vi "CTRE_Phoenix_CANifier_SetControlFramePeriod.vi"(8 "error in (no error)":errorcluster, 9 "periodMs":i32, 10 "Pigeon IMU Control Frame":T1=272384 items=["CondStatus_Control_1"=272384], 11 "PigeonIMUDevRef":T2={"DeviceStatus"={"status"=FALSE, "code"=0, "source"=""}, "Device Number"=0, "Type"=352321536, "Device ID"=0, "Handle"=0, "UsageFrame"=0, "Library Path"=path ""} {"Type" items=["CAN"=352321536, "TalonSRX"=33554432]}) -> (0 "error out":errorcluster, 3 "PigeonIMUDevRef":T2={"DeviceStatus"={"status"=FALSE, "code"=0, "source"=""}, "Device Number"=0, "Type"=352321536, "Device ID"=0, "Handle"=0, "UsageFrame"=0, "Library Path"=path ""} {"Type" items=["CAN"=352321536, "TalonSRX"=33554432]})   [LabVIEW 2017]
doc: "Set the period of the specified control frame."
uses:
  CTRE_PigeonIMU_DeviceRef.ctl
  CTRE_PigeonIMU_ConnectionType.ctl
  CTRE_PigeonIMU_ControlFrame.ctl
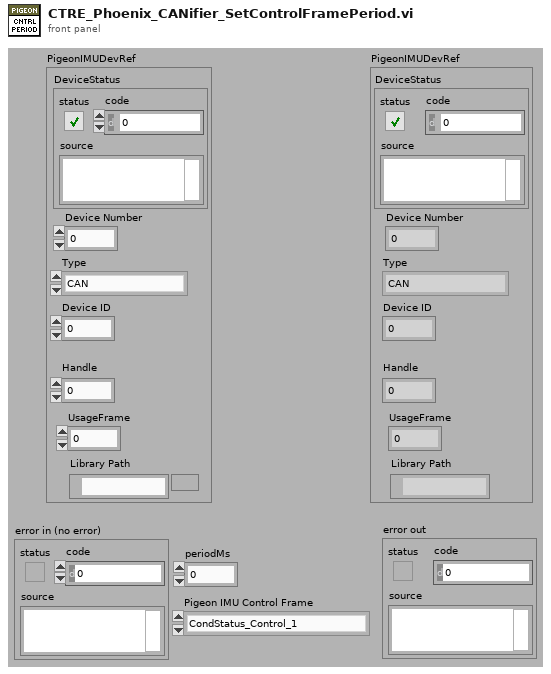
[diagram p1: front panel]
types:
  T1 = typedef "CTRE_PigeonIMU_ControlFrame.ctl" = u32
  T2 = typedef "CTRE_PigeonIMU_DeviceRef.ctl" = cluster{"DeviceStatus":errorcluster, "Device Number":u8, "Type":T3, "Device ID":u32, "Handle":u64, "UsageFrame":u32, "Library Path":path}
  T3 = typedef "CTRE_PigeonIMU_ConnectionType.ctl" = u32
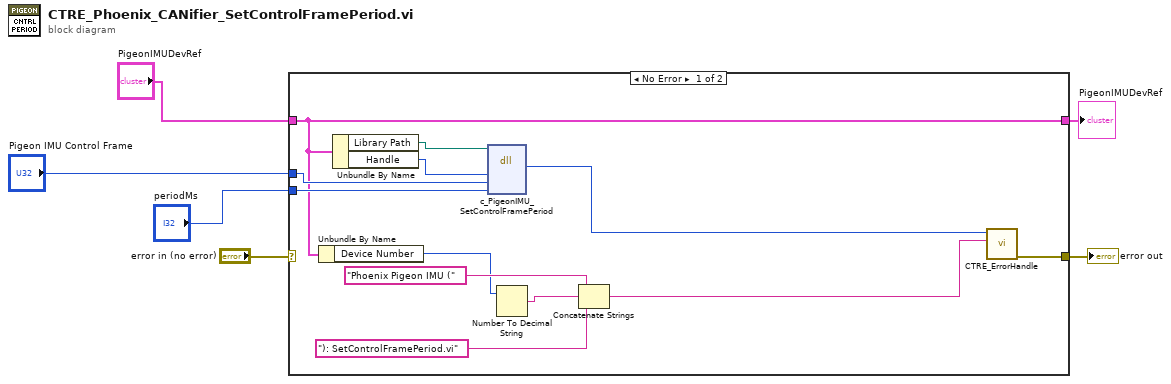
[diagram p0: block diagram]
diagram:
  n1 = case shown="No Error" "error in (no error)" {
    selector: "error in (no error)" -> [_ w20]
    tunnel: [w15 w20] -> w6
    tunnel: "PigeonIMUDevRef" -> [w9 w19]
    tunnel: [w9 w19] -> w2
    tunnel: "Pigeon IMU Control Frame" -> [w12 _]
    tunnel: "periodMs" -> [w11 _]
    frame No Error {
      n2 = Unbundle By Name(w9) -> ("Device Number"=w10:u8)
      n3 = Unbundle By Name(w9) -> ("Library Path"=w8:path, "Handle"=w7:u64)
      n4 = dll-call lib="?" fn="c_PigeonIMU_SetControlFramePeriod"(path in=w8, "handle"=w7, "frame"=w12, "periodMs"=w11) -> ("ErrorCode"=w13:i32)  [unwired: 5 in, 2 out]
      n5 = Number To Decimal String(number=w10) -> (decimal integer string=w17:string)  [unwired: 1 in]
      n6 = Concatenate Strings("Phoenix Pigeon IMU (" ("string"), w17, "): SetControlFramePeriod.vi" ("string")) -> (w14:string)
      n7 = call "CTRE_ErrorHandle.vi"("origin"=w14, "code"=w13) -> ("error out"=w15:errorcluster)  [unwired: 9 in]
    }
    frame Error {
    }
  }
  "error out" <- w6
  "PigeonIMUDevRef" <- w2
